vi "Monitor for Stop.vi"(8 "error in (no error)":errorcluster, 10 "service stop events":refnum<user-event>[](array[refnum]), 11 "Event Registration Refnum in":refnum<event-registration>) -> (0 "error out":errorcluster, 3 "Event Registration Refnum out":refnum<event-registration>)   [LabVIEW 2025, in "xnet_can_bus_monitor_api_server.lvlib"]
uses:
  xnet_can_bus_monitor_api_server.lvlib
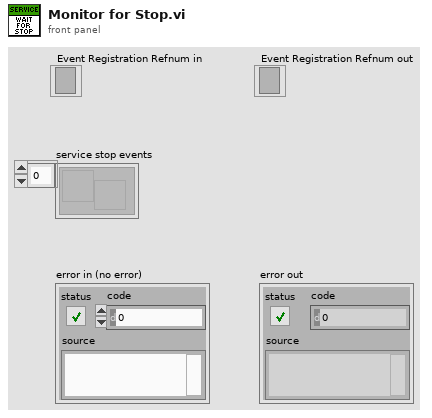
[diagram p1: front panel]
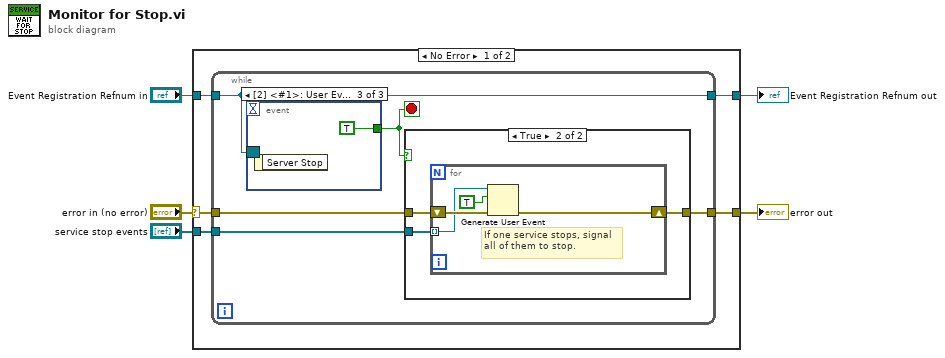
[diagram p0: block diagram]
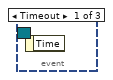
[diagram p3: hidden frame]
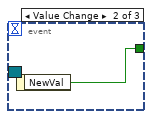
[diagram p4: hidden frame]
diagram:
  n1 = case shown="No Error" "error in (no error)" {
    selector: "error in (no error)" -> [w8 w27]
    tunnel: "Event Registration Refnum in" -> [w10 w26]
    tunnel: "service stop events" -> [w9 _]
    tunnel: [w6 w27] -> w5
    tunnel: [w7 w26] -> w4
    frame No Error {
      n2 = while {
        tunnel: w10 -> [w11]
        tunnel: [w11] -> w7
        tunnel: [w13] -> w6
        tunnel: w9 -> [w14]
        tunnel: w8 -> [w15]
        stop <- w12 stop-if-true
        n3 = event shown="[2] <#1>: User Event" {
          selector: w11 -> [_ _ _]
          dyn-events: _ -> [_ _ _]
          timeout: _ -> [_ _ _]
          tunnel: [_ w24 TRUE] -> w12
          event Timeout {
            n4 = event-data() -> ()  [unwired: 1 in, 1 out]
          }
          event Value Change {
            n5 = event-data() -> ("NewVal"=w24:bool)  [unwired: 1 in]
          }
          event User Event {
            n6 = event-data() -> ()  [unwired: 1 in, 1 out]
          }
        }
        n7 = case shown="True" w12 {
          tunnel: w15 -> [w16 w19]
          tunnel: w14 -> [_ w18]
          tunnel: [w16 w17] -> w13
          frame False {
          }
          frame True {
            n8 = for {
              shift-right: [w22] -> w17
              shift-left: w19 -> [w21]
              tunnel: w18 -> [w20] mode=indexing
              # "If one service stops, signal\nall of them to stop."
              n9 = Generate User Event(user event=w20, event data cluster=TRUE ("event data"), error in=w21) -> (error out=w22:errorcluster)  [unwired: 1 in, 1 out]
            }
          }
        }
      }
    }
    frame Error {
    }
  }
  "error out" <- w5
  "Event Registration Refnum out" <- w4
